vi "Get Valid Properties.vi"(8 "error in (no error)":errorcluster, 11 "Moving Ripple Noise in":refnum<class "Moving Ripple Noise.lvclass">) -> (0 "error out":errorcluster, 2 "Properties":string[](array[string]), 3 "Moving Ripple Noise out":refnum<class "Moving Ripple Noise.lvclass">)   [LabVIEW 2020, in "Moving Ripple Noise.lvclass"]
uses:
  Moving Ripple Noise.lvclass
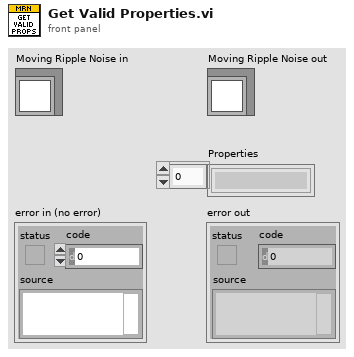
[diagram p1: front panel]
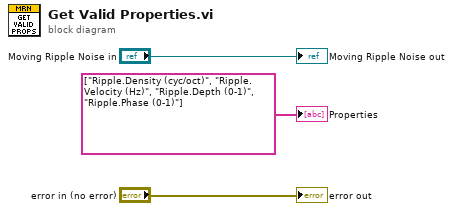
[diagram p0: block diagram]
diagram:
  "error out" <- "error in (no error)"
  "Moving Ripple Noise out" <- "Moving Ripple Noise in"
  "Properties" <- string[] ["Ripple.Density (cyc/oct)", "Ripple.Velocity (Hz)", "Ripple.Depth (0-1)", "Ripple.Phase (0-1)"] ("Properties")
